vi "Wire Between Unbundle And Bundle.vi"(8 "error in (no error)":errorcluster, 10 "Library ref in":refnum<vi>, 11 "VI Refnum":refnum<vi>) -> (0 "error IO":errorcluster, 2 "Library ref out":refnum<vi>, 3 "VI Refnum out":refnum<vi>)   [LabVIEW 2019, in "gRPC Template Creation Utility.lvlib"]
uses:
  gRPC Template Creation Utility.lvlib
  <vilib>/Utility/Data Type/NI_Data Type.lvlib
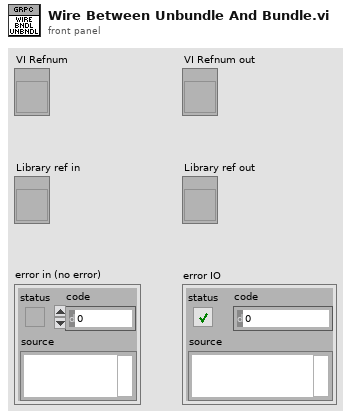
[diagram p1: front panel]
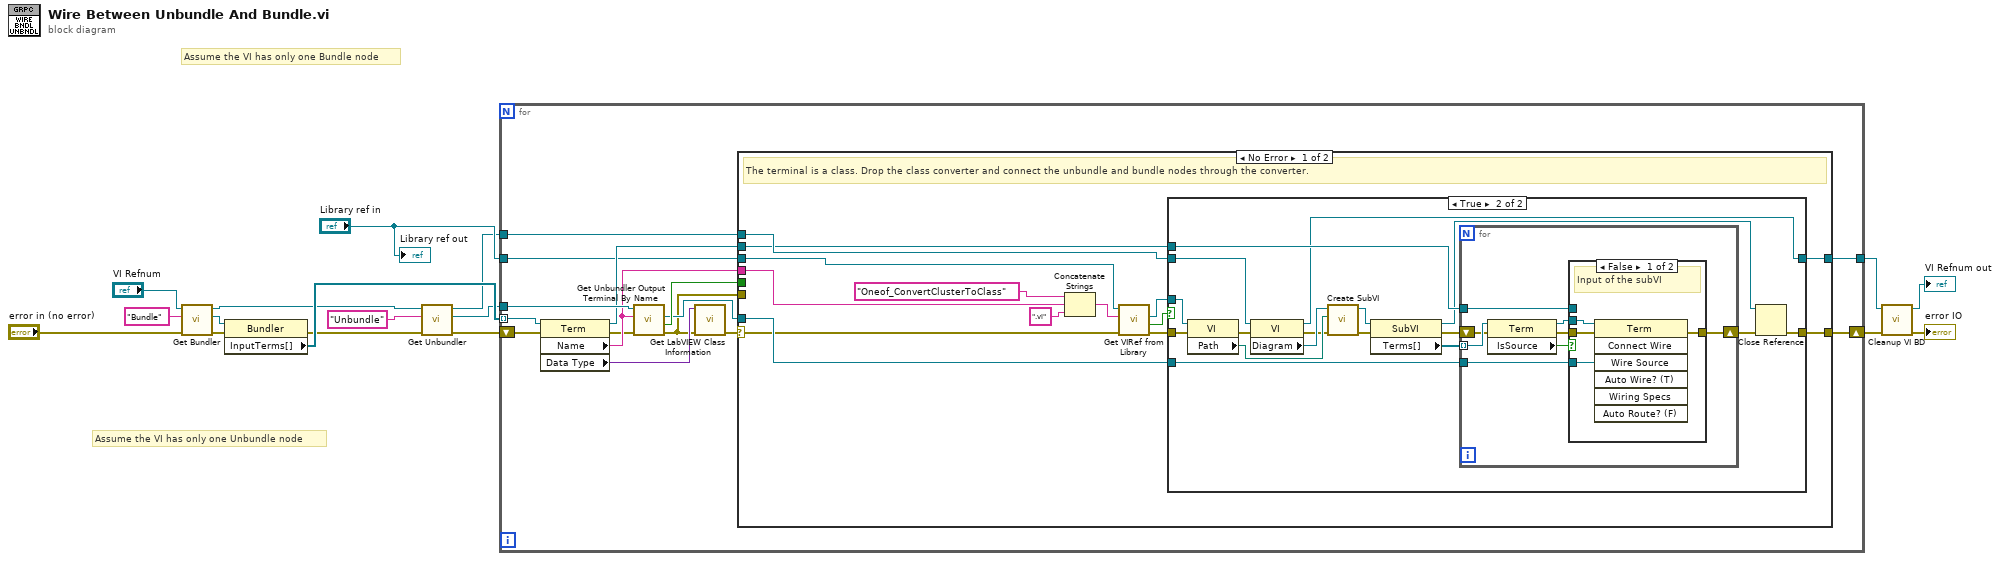
[diagram p0: block diagram]
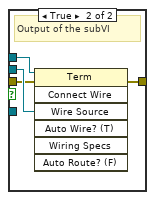
[diagram p3: hidden frame]
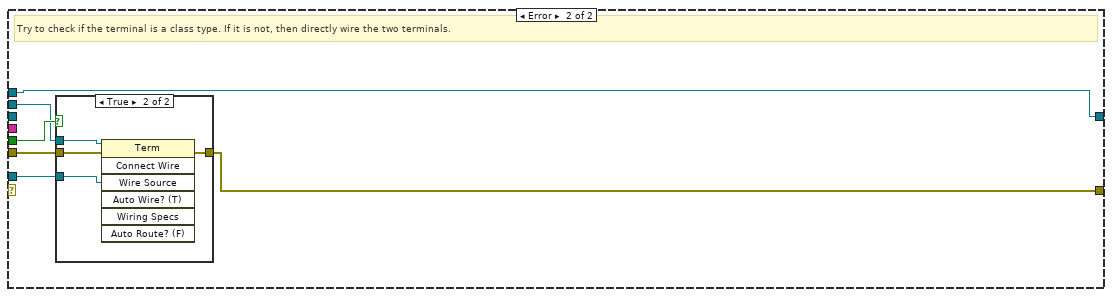
[diagram p4: hidden frame]
diagram:
  # "Assume the VI has only one Bundle node"
  # "Assume the VI has only one Unbundle node"
  n1 = call "Get Bundler.vi"("error in (no error)"="error in (no error)", "Label"="Bundle" ("Class Name"), "Owner VI in"="VI Refnum") -> ("error out"=w2:errorcluster, "Bundler ref out"=w11:refnum<vi>, "Owner VI out"=w3:refnum<vi>)  [unwired: 5 in, 1 out]
  n2 = property class="Bundler"(reference=w11, error in=w2) -> (error out=w1:errorcluster, "InputTerms[]"=w15:refnum<vi>[])  [unwired: 1 out]
  n3 = call "Get Unbundler.vi"("error in (no error)"=w1, "Label"="Unbundle" ("Class Name"), "Owner VI in"=w3) -> ("error out"=w5:errorcluster, "Unbundler Refnum"=w6:refnum<vi>, "Owner VI out"=w4:refnum<vi>)  [unwired: 5 in, 1 out]
  n4 = for {
    tunnel: w15 -> [w32] mode=indexing
    tunnel: w6 -> [w31]
    tunnel: "Library ref in" -> [w25]
    tunnel: w4 -> [w23]
    shift-right: [w21] -> w13
    shift-left: w5 -> [w19]
    tunnel: [w18] -> w14
    n5 = property class="Term"(reference=w32, error in=w19) -> (reference out=w28:refnum<vi>, error out=w22:errorcluster, "Name"=w24:string, "Data Type"=w27:variant)
    n6 = call "Get Unbundler Output Terminal By Name.vi"("error in (no error)"=w22, "Terminal name"=w24, "Unbundler in"=w31) -> ("error out"=w20:errorcluster, "Found?"=w30:bool, "Terminal Refnum"=w29:refnum<vi>)  [unwired: 5 in, 1 out]
    n7 = call <vilib>:"Get LabVIEW Class Information.vi"("error in (no error)"=w20, "variant"=w27) -> ("error out"=w26:errorcluster)  [unwired: 7 in, 2 out]
    n8 = case shown="No Error" w26 {
      selector: w26 -> [w36 _]
      tunnel: w30 -> [_ w87]
      tunnel: w29 -> [w38 w86]
      tunnel: w28 -> [w37 w85]
      tunnel: w25 -> [w46 _]
      tunnel: w24 -> [w44 _]
      tunnel: w23 -> [w39 w82]
      tunnel: [w34 w83] -> w21
      tunnel: w20 -> [_ w84]
      tunnel: [w33 w82] -> w18
      frame No Error {
        # "The terminal is a class. Drop the class converter and connect the unbundle and bundle nodes through the converter."
        n9 = Concatenate Strings("Oneof_ConvertClusterToClass" ("string"), w44, ".vi" ("string")) -> (w42:string)
        n10 = call "Get VIRef from Library.vi"("error in (no error)"=w36, "Item Name"=w42, "Library"=w46) -> ("error out"=w35:errorcluster, "Found ?"=w41:bool, "VIref out"=w40:refnum<vi>)  [unwired: 5 in, 1 out]
        n11 = case shown="True" w41 {
          tunnel: w40 -> [_ w65]
          tunnel: w39 -> [w47 w63]
          tunnel: w38 -> [_ w58]
          tunnel: w37 -> [_ w57]
          tunnel: w35 -> [w48 w54]
          tunnel: [w48 w50] -> w34
          tunnel: [w47 w49] -> w33
          frame False {
          }
          frame True {
            n12 = property class="VI"(reference=w65, error in=w54) -> (error out=w56:errorcluster, "Path"=w64:path)  [unwired: 1 out]
            n13 = property class="VI"(reference=w63, error in=w56) -> (reference out=w49:refnum<vi>, error out=w55:errorcluster, "Diagram"=w62:refnum<vi>)
            n14 = call "Create SubVI.vi"("error in (no error)"=w55, "Path"=w64, "Diagram in"=w62) -> ("error out"=w60:errorcluster, "subVI refnum"=w61:refnum<vi>)  [unwired: 7 in]
            n15 = property class="SubVI"(reference=w61, error in=w60) -> (reference out=w52:refnum<vi>, error out=w53:errorcluster, "Terms[]"=w59:refnum<vi>[])
            n16 = for {
              tunnel: w59 -> [w73] mode=indexing
              tunnel: w58 -> [w70]
              tunnel: w57 -> [w69]
              shift-right: [w66] -> w51
              shift-left: w53 -> [w68]
              n17 = property class="Term"(reference=w73, error in=w68) -> (reference out=w71:refnum<vi>, error out=w67:errorcluster, "IsSource"=w72:bool)
              n18 = case shown="False" w72 {
                tunnel: w71 -> [w77 w81]
                tunnel: w70 -> [w76 _]
                tunnel: w69 -> [_ w80]
                tunnel: w67 -> [w75 w79]
                tunnel: [w74 w78] -> w66
                frame False {
                  # "Input of the subVI"
                  n19 = invoke class="Term" method="Connect Wire"(reference=w77, error in=w75, "Wire Source"=w76) -> (error out=w74:errorcluster)  [unwired: 4 in, 6 out]
                }
                frame True {
                  # "Output of the subVI"
                  n20 = invoke class="Term" method="Connect Wire"(reference=w80, error in=w79, "Wire Source"=w81) -> (error out=w78:errorcluster)  [unwired: 4 in, 6 out]
                }
              }
            }
            n21 = Close Reference(reference=w52, error in (no error)=w51) -> (error out=w50:errorcluster)
          }
        }
      }
      frame Error {
        # "Try to check if the terminal is a class type. If it is not, then directly wire the two terminals."
        n22 = case shown="True" w87 {
          tunnel: w86 -> [_ w91]
          tunnel: w85 -> [_ w92]
          tunnel: w84 -> [w88 w90]
          tunnel: [w88 w89] -> w83
          frame False {
          }
          frame True {
            n23 = invoke class="Term" method="Connect Wire"(reference=w92, error in=w90, "Wire Source"=w91) -> (error out=w89:errorcluster)  [unwired: 4 in, 6 out]
          }
        }
      }
    }
  }
  n24 = call "Cleanup VI BD.vi"("error in (no error)"=w13, "VI in"=w14) -> ("error out"=→"error IO":errorcluster, "VI out"=→"VI Refnum out":refnum<vi>)  [unwired: 8 in]
  "Library ref out" <- "Library ref in"
